vi "sync and trig.vi"(8 "error in (no error)":errorcluster, 11 "p2p vst in":refnum<class "p2p vst.lvclass">) -> (0 "error out":errorcluster, 3 "p2p vst out":refnum<class "p2p vst.lvclass">)   [LabVIEW 2021, in "p2p vst.lvclass"]
uses:
  p2p vst.lvclass
  p2p vst.lvclass/p2p vst.ctl
  <vilib>/rvi/interface/nirviReadWriteControl/nirviReadWriteControl.xnode
  NiFpgaLv.dll
  <vilib>/Utility/error.llb/Error Cluster From Error Code.vi
  <vilib>/rvi/interface/Simulation/niFpgaSimulationCallBeginRW.vi
  <vilib>/rvi/errors/niLvFpgaAdjustHostInterfaceError.vi
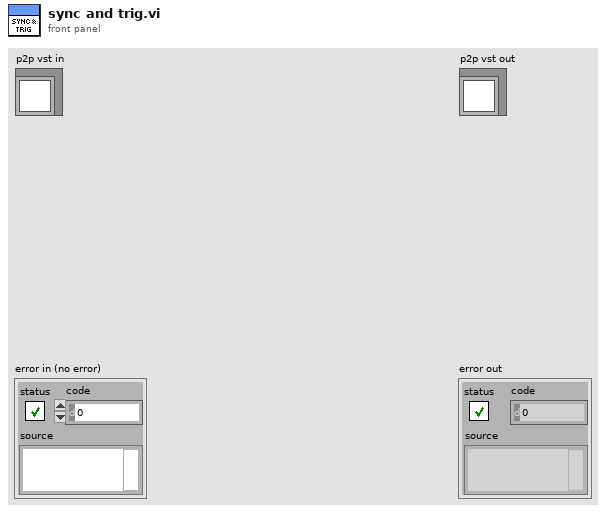
[diagram p1: front panel]
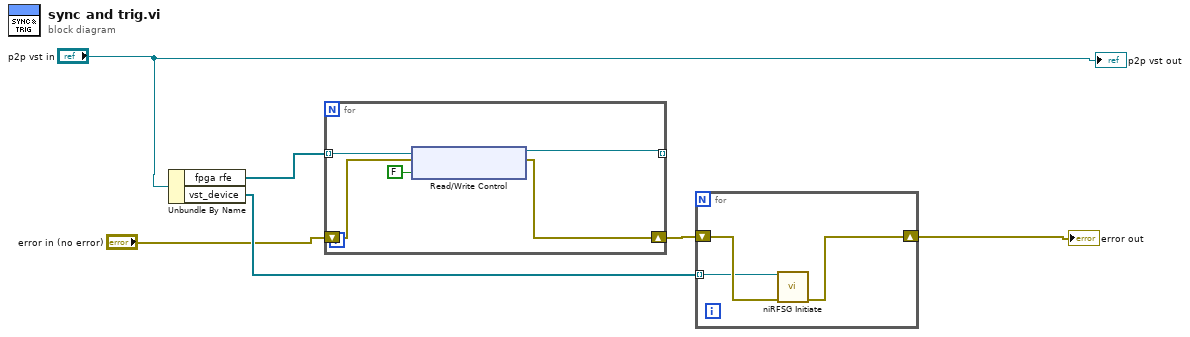
[diagram p0: block diagram]
diagram:
  n1 = Unbundle By Name("p2p vst in") -> ("fpga rfe"=w6:refnum<k20>[], "vst_device"=w4:refnum<k15>[])
  n2 = for {
    tunnel: w6 -> [w11] mode=indexing
    tunnel: [w10] -> _ mode=indexing
    shift-right: [w7] -> w5
    shift-left: "error in (no error)" -> [w9]
    n3 = xnode "Read/Write Control"("FPGA VI Reference In"=w11, "error in"=w9, "reset system clock"=FALSE) -> ("FPGA VI Reference Out"=w10:refnum<k20>, "error out"=w7:errorcluster)
  }
  n4 = for {
    shift-right: [w13] -> w1
    shift-left: w5 -> [w14]
    tunnel: w4 -> [w12] mode=indexing
    n5 = call <instrlib>:"niRFSG Initiate.vi"("instrument handle"=w12, "error in"=w14) -> ("error out"=w13:errorcluster)  [unwired: 12 in, 1 out]
  }
  "error out" <- w1
  "p2p vst out" <- "p2p vst in"
